vi "Debug - Verbose - Append Error Handler Text to File.vi"(11 "Strings to Append":string[](array[string])) -> ()   [LabVIEW 2017, in "Communications Library.lvlib"]
doc: "Appends an array of strings to the end of a debug file.\n\nNote:\nThe error wires have been purposefuly excluded from this VI. The text should be appended to the debug file, regardless of the error state.\nThis VI must be non-reentrant. Setting this VI to reentrant execution can cause multiple threads to attempt simulatneous write access to the same file, causing a crash."
uses:
  Communications Library.lvlib
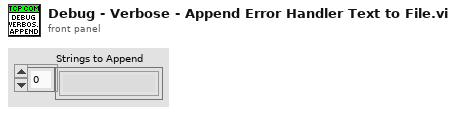
[diagram p1: front panel]
types:
  T1 = enum16{"open", "replace", "create", "open or create", "replace or create", "replace or create with confirmation"}
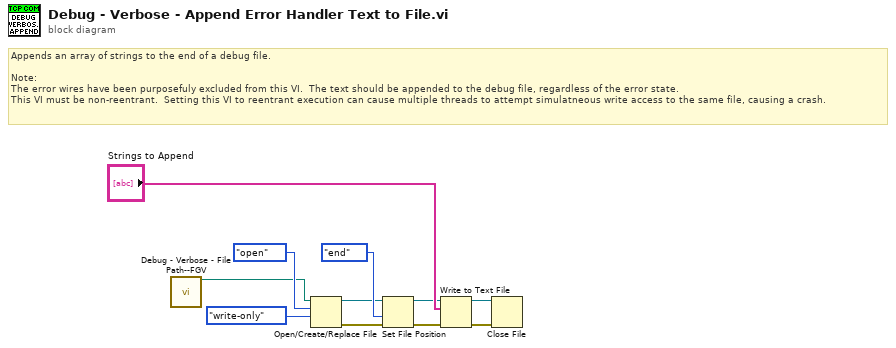
[diagram p0: block diagram]
diagram:
  # "Appends an array of strings to the end of a debug file.\n\nNote:\nThe error wires have been purposefuly excluded from this VI.  The text should be appended to the debug file, regardless of the error state.\nThis VI must be non-reentrant.  Setting this VI to reentrant execution can cause multiple threads to attempt simulatneous write access to the same file, causing a crash."
  n1 = call "Debug - Verbose - File Path--FGV.vi"() -> ("Debug Pathname"=w1:path)  [unwired: 11 in]
  n2 = Open/Create/Replace File(file path (use dialog)=w1, operation (0:open)=T1."open", access (0:read/write)=enum16{"read/write", "read-only", "write-only"}."write-only") -> (refnum out=w4:refnum<file>, error out=w5:errorcluster)  [unwired: 3 in, 1 out]
  n3 = Set File Position(refnum=w4, from (0:start)=enum16{"start", "end", "current"}."end", error in=w5) -> (refnum out=w8:refnum<file>, error out=w6:errorcluster)  [unwired: 1 in]
  n4 = Write to Text File(file (use dialog)=w8, text="Strings to Append", error in=w6) -> (refnum out=w11:refnum<file>, error out=w10:errorcluster)  [unwired: 1 in, 1 out]
  n5 = Close File(refnum=w11, error in=w10) -> ()  [unwired: 2 out]
